vi "cost_complexity_pruning_path.vi"(8 "error in (no error)":errorcluster caption="entrée d'erreur (pas d'erreur)", 11 "Tree.lvclass":refnum<class "Tree.lvclass">) -> (0 "error out":errorcluster caption="sortie d'erreur", 2 "out":cluster{"ccp_alphas":dbl[], "impurities":dbl[]}, 3 "Tree.lvclass 2":refnum<class "Tree.lvclass">)   [LabVIEW 2020, in "Tree.lvclass"]
doc: "Compute the pruning path during Minimal Cost-Complexity Pruning.\n\n See :ref:`minimal_cost_complexity_pruning` for details on the pruning\n process.\n\n Parameters\n ----------\n X : {array-like, sparse matrix} of shape (n_samples, n_features)\n The training input samples. Internally, it will be converted to\n ``dtype=np.float32`` and if a sparse matrix is provided\n to a sparse ``csc_matrix``.\n\n y : array-like of shape (n_samples,) or (n_samples, n_outputs)\n The target values (class labels) as integers or strings.\n\n sample_weight : array-like of shape (n_samples,), default=None\n Sample weights. If None, then samples are equally weighted. Splits\n that would create child nodes with net zero or negative weight are\n ignored while searching for a split in each node. Splits are also\n ignored if they would result in any single class carrying a\n negative weight in either child node.\n\n Returns\n -------\n ccp_path : :class:`~sklearn.utils.Bunch`\n Dictionary-like object, with the following attributes.\n\n ccp_alphas : ndarray\n Effective alphas of subtree during pruning.\n\n impurities : ndarray\n Sum of the impurities of the subtree leaves for the\n corresponding alpha value in ``ccp_alphas``."
uses:
  Tree.lvclass
  C:/Users/cipop/TDF Dropbox/2_Technologies de France/1 - Services et Etudes/PLAIY/2 - DEV/PLAIYLAB/code/Python/Python.lvclass
  C:/Users/cipop/TDF Dropbox/2_Technologies de France/1 - Services et Etudes/PLAIY/2 - DEV/PLAIYLAB/code/Model/Model.lvclass
  Tree.lvclass/Tree.ctl
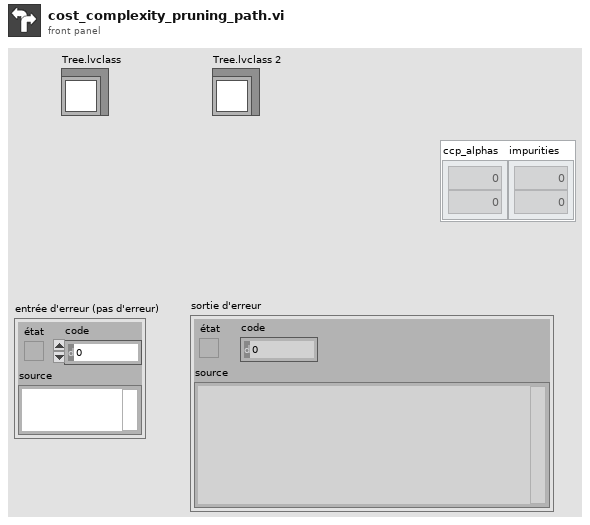
[diagram p1: front panel]
types:
  T1 = typedef "data.ctl" = cluster{"name":string, "X":dbl[][]}
  T2 = typedef "tree_data.ctl" = cluster{"y":dbl[][], "sample_weight":dbl[], "check_input":bool}
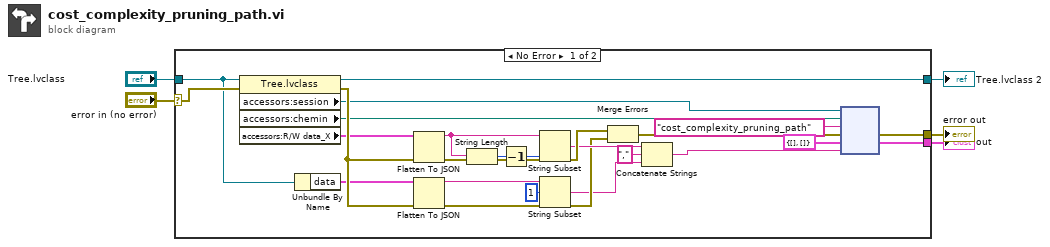
[diagram p0: block diagram]
diagram:
  n1 = case shown="No Error" "error in (no error)" {
    selector: "error in (no error)" -> [w27 w31]
    tunnel: [w28 w31] -> w2
    tunnel: [w8 w30] -> w3
    tunnel: "Tree.lvclass" -> [w11 w30]
    tunnel: [w13 _] -> w1
    frame No Error {
      n2 = property class="Tree.lvclass"(reference=w11, error in=w27) -> (reference out=w8:refnum<class "Tree.lvclass">, error out=w18:errorcluster, "accessors:session"=w7:refnum<k35>, "accessors:chemin"=w6:path, "accessors:R/W data_X"=w12:T1)
      n3 = Unbundle By Name(w11) -> ("data"=w10:T2)
      n4 = Flatten To JSON(anything=w12, error in (no error)=w18) -> (JSON string=w24:string, 11:w21:errorcluster)  [unwired: 1 in]
      n5 = Flatten To JSON(anything=w10, error in (no error)=w18) -> (JSON string=w22:string, 11:w17:errorcluster)  [unwired: 1 in]
      n6 = String Length(string=w24) -> (length=w26:i32)
      n7 = Decrement(x=w26) -> (x-1=w25:i32)
      n8 = String Subset(string=w24, length (rest)=w25) -> (substring=w20:string)  [unwired: 1 in]
      n9 = String Subset(string=w22, offset (0)=1) -> (substring=w15:string)  [unwired: 1 in]
      n10 = Merge Errors(w21, w17) -> (w9:errorcluster)
      n11 = Concatenate Strings(w20, "," ("string"), w15) -> (w19:string)
      n12 = node(w7, w6, "cost_complexity_pruning_path" ("nom de la fonction"), w9, cluster{"ccp_alphas":dbl[], "impurities":dbl[]} {"ccp_alphas"=[], "impurities"=[]} ("out"), w19) -> (w28:errorcluster, w13:cluster{"ccp_alphas":dbl[], "impurities":dbl[]})  [unwired: 1 in, 3 out]
    }
    frame Error {
    }
  }
  "error out" <- w2
  "Tree.lvclass 2" <- w3
  "out" <- w1
